vi "Report_Type.vi"(8 "error in (no error)":errorcluster, 11 "IB_PackedLib in":refnum<class "IB_PackedLib.lvclass">) -> (0 "error out":errorcluster, 2 "type":string, 3 "IB_PackedLib out":refnum<class "IB_PackedLib.lvclass">)   [LabVIEW 2020, in "IB_PackedLib.lvclass"]
uses:
  <vilib>/AppBuilder/IB_Classes/Source/Container/Build/PackedLib/IB_PackedLib.lvclass
  <vilib>/AppBuilder/IB_Classes/Source/Container/Build/PackedLib/IB_PackedLib.lvclass/IB_PackedLib.ctl
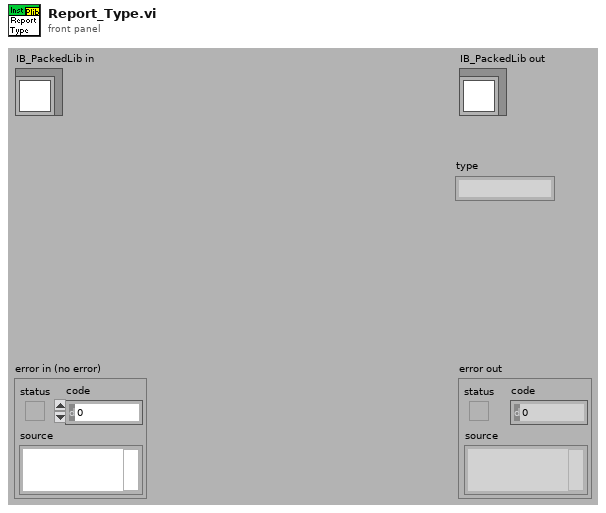
[diagram p1: front panel]
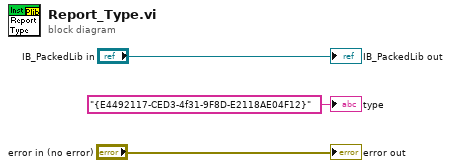
[diagram p0: block diagram]
diagram:
  "error out" <- "error in (no error)"
  "IB_PackedLib out" <- "IB_PackedLib in"
  "type" <- "{E4492117-CED3-4f31-9F8D-E2118AE04F12}" ("type")
